vi "Load Core.vi"(0 "Class Loader in":refnum<class "Class Loader.lvclass">, 5 "Caller Enqueuer":refnum<class "Message Enqueuer.lvclass">, 7 "Reference Class Path":path, 9 "Class Relative Paths Path":path, 11 "error in (no error)":errorcluster) -> (4 "Class Loader out":refnum<class "Class Loader.lvclass">, 15 "error out":errorcluster)   [LabVIEW 2023, in "Class Loader.lvlib" / "Class Loader.lvclass"]
uses:
  Class Loader.lvclass
  <vilib>/ActorFramework/Message Enqueuer/Message Enqueuer.lvclass
  Class Loader Interfaces/Class Loader Interfaces Messages/Class Loading Result Msg/Class Loading Result Msg.lvclass/Class Loading Result Msg.ctl
  <vilib>/ActorFramework/Message Enqueuer/Message Enqueuer.lvclass/Message Enqueuer.ctl
  <vilib>/ActorFramework/Report Error Msg/Report Error Msg.lvclass/Report Error Msg.ctl
  e0b067aa-0a6b-4c0e-95c6-395db7073fd2.vi/b0178052-0c48-4c9a-874f-40b592e34ac5.vi
  <vilib>/ActorFramework/Message Enqueuer/Enqueue.vi
  Class Loader Interfaces/Class Loader Interfaces Messages/Class Loading Result Msg/Class Loading Result Msg.lvclass
  <vilib>/ActorFramework/Report Error Msg/Report Error Msg.lvclass
  <vilib>/Utility/LVClass/Get LV Class Name.vi
  <resource>/AFDebug/Generate Trace for Message.vi
  <vilib>/ActorFramework/Message Priority Queue/Priority Enqueue.vi
  Class Loader.lvclass/Class Loader.ctl
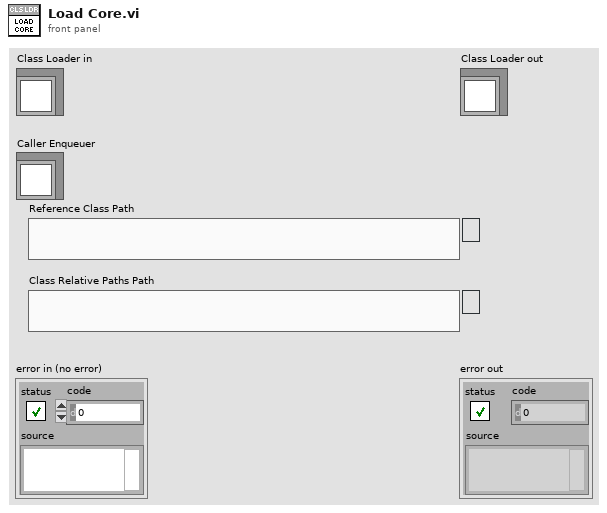
[diagram p1: front panel]
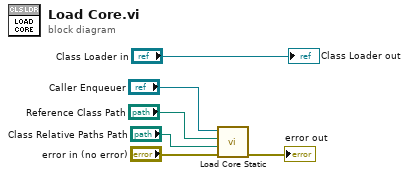
[diagram p0: block diagram]
diagram:
  n1 = call "Load Core Static.vi"("error in (no error)"="error in (no error)", "Class Relative Paths Path"="Class Relative Paths Path", "Reference Class Path"="Reference Class Path", "Message Enqueuer in"="Caller Enqueuer") -> ("error out"=→"error out":errorcluster)  [unwired: 7 in]
  "Class Loader out" <- "Class Loader in"
